vi "Conectando máquinas con Zerotier 1.vi"() -> ()   [LabVIEW 2019]
panel:
  in  "stop":bool
  out "connection ID 2":refnum<k5>
  out "connection ID":refnum<k5>
  in  "Datos a enviar":string
  in  "Datos recibidos":string
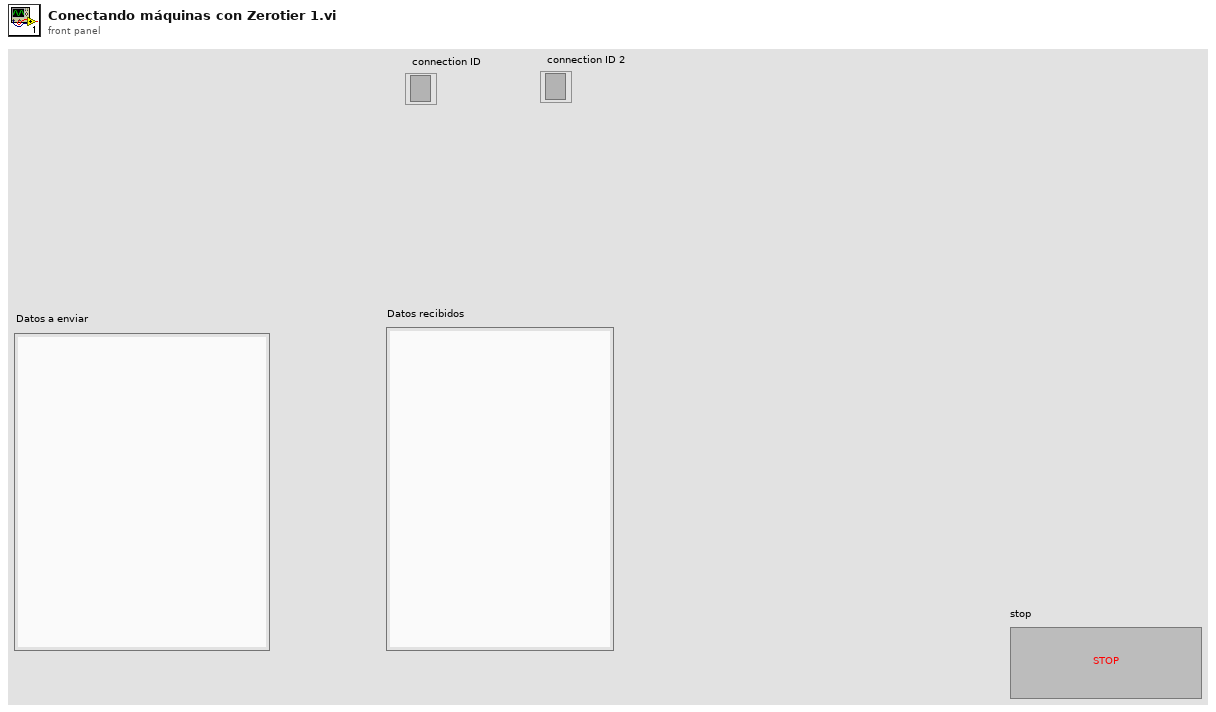
[diagram p1: front panel]
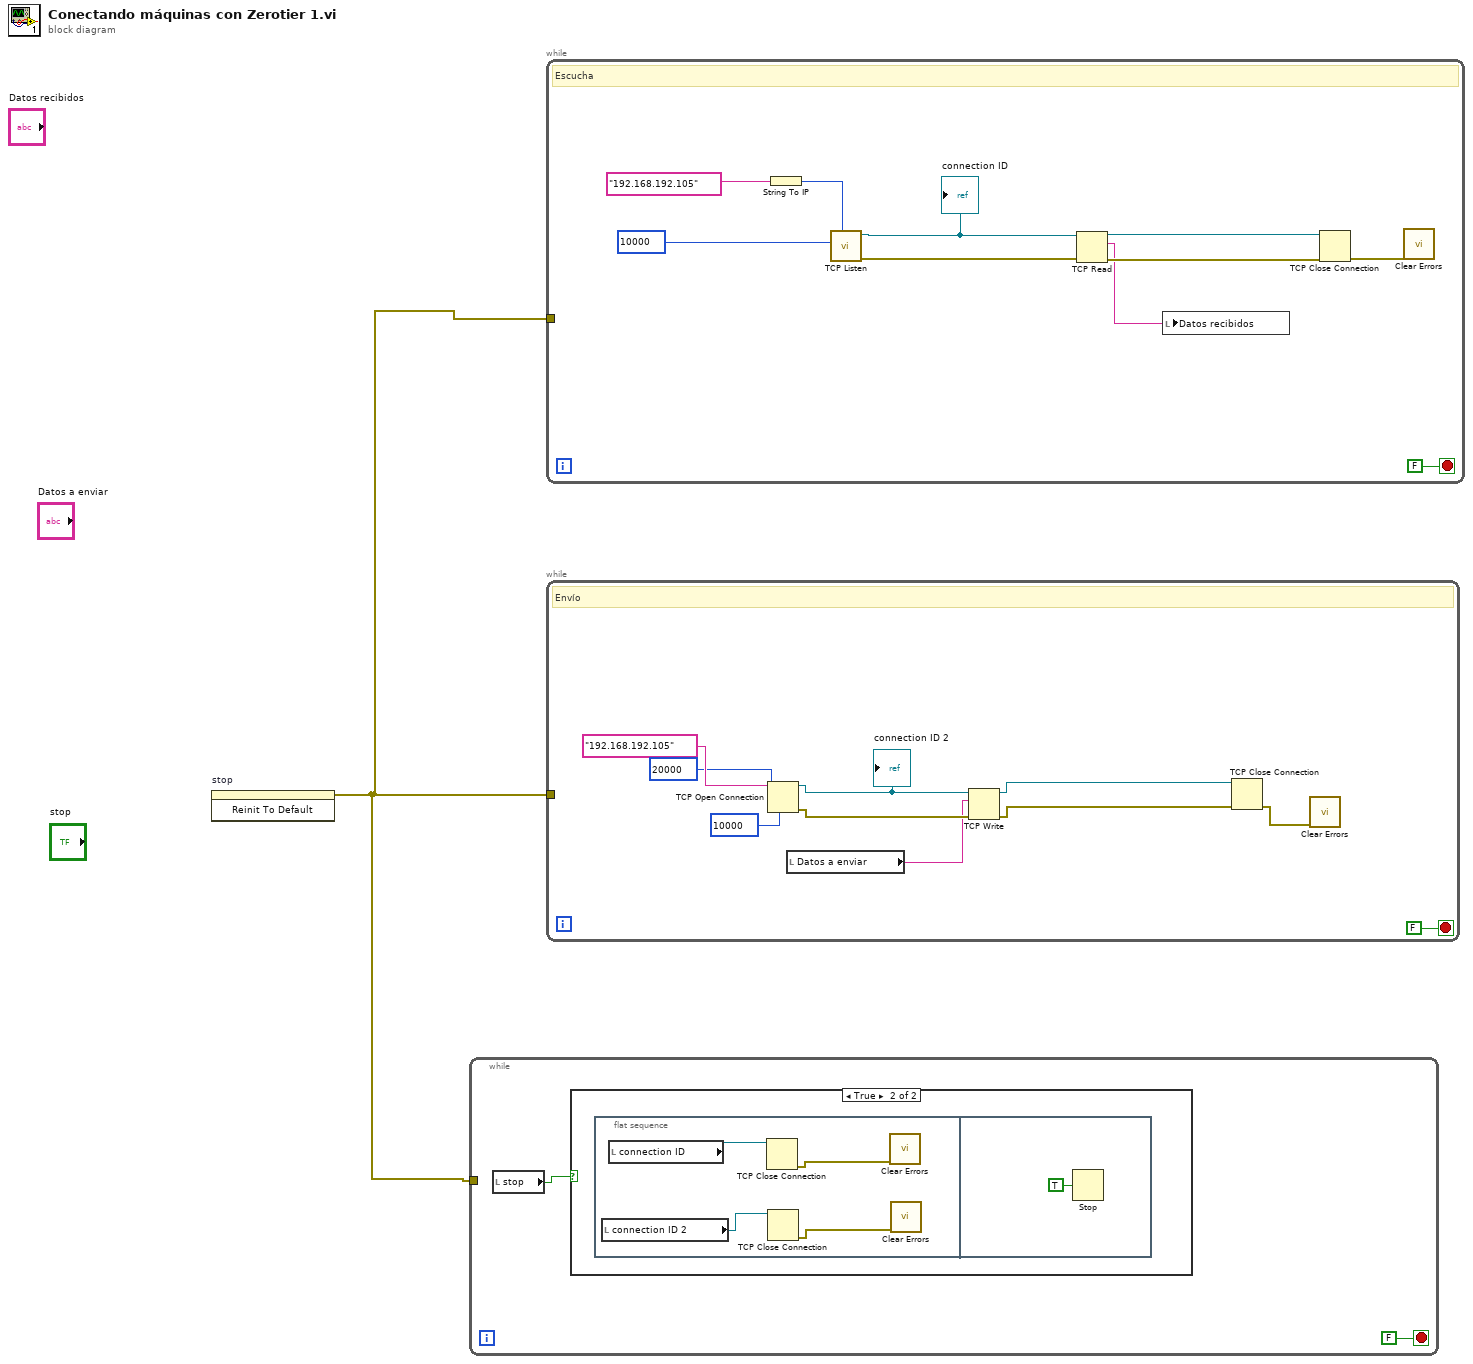
[diagram p0: block diagram]
diagram:
  n1 = invoke on="stop" class="Bool (strict)" method="Reinit To Default"() -> (error out=w1:errorcluster)  [unwired: 3 in, 2 out]
  n2 = while {
    tunnel: w1 -> [_]
    stop <- FALSE stop-if-true
    n3 = local read "stop"() -> (w2:bool)
    n4 = case shown="True" w2 {
      frame False {
      }
      frame True {
        n5 = flat-sequence {
          frame #0 {
            n6 = local read "connection ID 2"() -> (w6:refnum<k5>)
            n7 = local read "connection ID"() -> (w7:refnum<k5>)
            n8 = TCP Close Connection(connection ID=w7) -> (error out=w5:errorcluster)  [unwired: 2 in, 1 out]
            n9 = TCP Close Connection(connection ID=w6) -> (error out=w4:errorcluster)  [unwired: 2 in, 1 out]
            n10 = call <vilib>:"Clear Errors.vi"("error in (no error)"=w5) -> ()  [unwired: 5 in, 2 out]
            n11 = call <vilib>:"Clear Errors.vi"("error in (no error)"=w4) -> ()  [unwired: 5 in, 2 out]
          }
          frame #1 {
            n12 = Stop(stop? (T)=TRUE) -> ()
          }
        }
      }
    }
  }
  n13 = while {
    tunnel: w1 -> [_]
    stop <- FALSE stop-if-true
    # "Escucha"
    n14 = String To IP(1:"192.168.192.105" ("name")) -> (0:w17:u32)
    n15 = call <vilib>:"TCP Listen.vi"("net address"=w17, "port"=u16 10000) -> ("error out"=w13:errorcluster, "connection ID"=w15:refnum<k5>)  [unwired: 5 in, 3 out]
    "connection ID" <- w15
    n16 = TCP Read(connection ID=w15, error in (no error)=w13) -> (connection ID out=w14:refnum<k5>, data out=w11:string, error out=w12:errorcluster)  [unwired: 3 in]
    n17 = local write "Datos recibidos"(w11) -> ()
    n18 = TCP Close Connection(connection ID=w14, error in (no error)=w12) -> (error out=w9:errorcluster)  [unwired: 1 in, 1 out]
    n19 = call <vilib>:"Clear Errors.vi"("error in (no error)"=w9) -> ()  [unwired: 5 in, 2 out]
  }
  n20 = while {
    tunnel: w1 -> [_]
    stop <- FALSE stop-if-true
    # "Envío"
    n21 = TCP Open Connection(address="192.168.192.105", remote port or service name=u16 20000, local port=u16 10000 ("local port (0)")) -> (connection ID=w23:refnum<k5>, error out=w25:errorcluster)  [unwired: 2 in]
    "connection ID 2" <- w23
    n22 = local read "Datos a enviar"() -> (w21:string)
    n23 = TCP Write(connection ID=w23, data in=w21, error in (no error)=w25) -> (connection ID out=w22:refnum<k5>, error out=w24:errorcluster)  [unwired: 1 in, 1 out]
    n24 = TCP Close Connection(connection ID=w22, error in (no error)=w24) -> (error out=w19:errorcluster)  [unwired: 1 in, 1 out]
    n25 = call <vilib>:"Clear Errors.vi"("error in (no error)"=w19) -> ()  [unwired: 5 in, 2 out]
  }
